vi "RonLinear.vi"(0 "refnum":refnum<file>) -> (4 "refnum out":refnum<file>, 6 "# lines per scan":i32, 8 "sample rate":u16, 10 "# rf points per line":u16, 13 "Scan Settings":T1 {"prf (kHz)" format="%.2f"; "Gain (db)" items=["26.0", "40.0", "54.0"]; "LP Filt (MHz)" items=["20", "50", "100", "200"]; "HP Filt(KHz)" items=["1", "1000", "3000", "10000"]; "Damping (In Ohm)" items=["7", "10", "16", "20", "26", "30", "40", "50"]; "Energy (microJ)" items=["1", "2", "4", "8", "16", "32"]}, 14 "Patient Info":T2={"ID"="", "extended ID"="", "age"=0, "sex"="", "previously\nscanned"="N", "PSA"=0.0, "LOS"=1, "Ethnicty"=3} {"Ethnicty" items=["Am Ind or Alaska", "Asian, Pac Islander", "Black, not Hispanic", "Hispanic", "White, not hispanic", "other, unknown"]; "LOS" items=["1", "2", "3", "4", "5"]; "PSA" format="%.1f"}, 15 "A/D info":T3={"# rf points per line"=0, "# lines per scan"=0, "sample rate MHz"=0, "# A/D bits"=8, "# bytes per A/D"=1, "TGC Flag"=0, "A/D Type"=""})   [LabVIEW 2022 SP3]
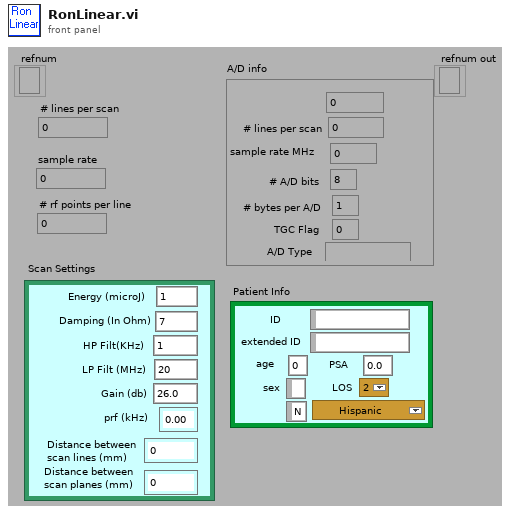
[diagram p1: front panel]
types:
  T1 = cluster{"Energy (microJ)":u8, "Damping (In Ohm)":u8, "HP Filt(KHz) ":u8, "LP Filt (MHz)":u8, "Gain (db)":u8, "prf (kHz)":sgl, "Distance between\nscan lines (mm)":u16, "Distance between\nscan planes (mm)":u16}
  T2 = cluster{"ID":string, "extended ID":string, "age":u16, "sex":string, "previously\nscanned":string, "PSA":sgl, "LOS":u8, "Ethnicty":u8}
  T3 = cluster{"# rf points per line":u16, "# lines per scan":u16, "sample rate MHz":u16, "# A/D bits":i16, "# bytes per A/D":u16, "TGC Flag":u16, "A/D Type":string}
  T4 = cluster{"Energy (microJ)":u8, "Damping (In Ohm)":u8, "HP Filt(KHz)":u8, "LP Filt (MHz)":u8, "Gain (db)":u8, "prf (kHz)":sgl, "Distance between\nscan lines (mm)":u16, "Distance between\nscan planes (mm)":u16}
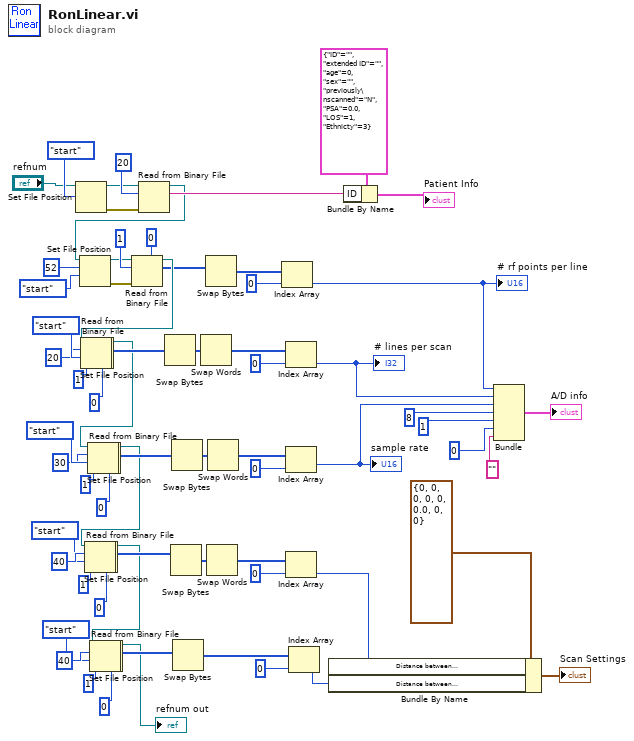
[diagram p0: block diagram]
diagram:
  n1 = Set File Position(refnum="refnum", from (0:start)=enum16{"start", "end", "current"}."start" ("pos mode (0:2)")) -> (refnum out=w7:refnum<file>, error out=w6:errorcluster)  [unwired: 1 in, 1 out]
  n2 = Read from Binary File(8:w6, 10:20, 11:w7) -> (2:w52:string, 3:w44:refnum<file>)  [unwired: 5 out]
  n3 = Set File Position(offset (in bytes) (0)=52 ("pos offset (0)"), refnum=w44, from (0:start)=enum16{"start", "end", "current"}."start" ("pos mode (0:2)")) -> (refnum out=w9:refnum<file>, error out=w8:errorcluster)  [unwired: 1 in]
  n4 = Read from Binary File(5:i16 0, 8:w8, 10:1 ("count"), 11:w9) -> (2:w42:i16[], 3:w43:refnum<file>)  [unwired: 4 out]
  n5 = Set File Position(offset (in bytes) (0)=20 ("pos offset (0)"), refnum=w43, from (0:start)=enum16{"start", "end", "current"}."start" ("pos mode (0:2)")) -> (refnum out=w3:refnum<file>, error out=w2:errorcluster)  [unwired: 1 in]
  n6 = Read from Binary File(5:0, 8:w2, 10:1 ("count"), 11:w3) -> (2:w71:i32[], 3:w58:refnum<file>)  [unwired: 4 out]
  n7 = Set File Position(offset (in bytes) (0)=30 ("pos offset (0)"), refnum=w58, from (0:start)=enum16{"start", "end", "current"}."start" ("pos mode (0:2)")) -> (refnum out=w5:refnum<file>, error out=w4:errorcluster)  [unwired: 1 in]
  n8 = Read from Binary File(5:0, 8:w4, 10:1 ("count"), 11:w5) -> (2:w63:i32[], 3:w33:refnum<file>)  [unwired: 4 out]
  n9 = Set File Position(offset (in bytes) (0)=40 ("pos offset (0)"), refnum=w33, from (0:start)=enum16{"start", "end", "current"}."start" ("pos mode (0:2)")) -> (refnum out=w11:refnum<file>, error out=w10:errorcluster)  [unwired: 1 in]
  n10 = Read from Binary File(5:0, 8:w10, 10:1 ("count"), 11:w11) -> (2:w28:i32[], 3:w19:refnum<file>)  [unwired: 4 out]
  n11 = Set File Position(offset (in bytes) (0)=40 ("pos offset (0)"), refnum=w19, from (0:start)=enum16{"start", "end", "current"}."start" ("pos mode (0:2)")) -> (refnum out=w13:refnum<file>, error out=w12:errorcluster)  [unwired: 1 in]
  n12 = Read from Binary File(5:i16 0, 8:w12, 10:1 ("count"), 11:w13) -> (2:w20:i16[], 3:→"refnum out":refnum<file>)  [unwired: 4 out]
  n13 = Swap Bytes(anything=w71) -> (byte swapped=w68:i32[])
  n14 = Swap Bytes(anything=w28) -> (byte swapped=w30:i32[])
  n15 = Swap Bytes(anything=w63) -> (byte swapped=w60:i32[])
  n16 = Swap Bytes(anything=w20) -> (byte swapped=w18:i16[])
  n17 = Swap Words(1:w68) -> (0:w67:i32[])
  n18 = Swap Bytes(anything=w42) -> (byte swapped=w40:i16[])
  n19 = Swap Words(1:w30) -> (0:w29:i32[])
  n20 = Swap Words(1:w60) -> (0:w59:i32[])
  n21 = Index Array(array=w40, index=0) -> (element=w14:i16)
  "# rf points per line" <- w14
  n22 = Index Array(array=w67, index=0) -> (element=w56:i32)
  "# lines per scan" <- w56
  n23 = Index Array(array=w59, index=0) -> (element=w57:i32)
  "sample rate" <- w57
  n24 = Index Array(array=w29, index=0) -> (element=w16:i32)
  n25 = Index Array(array=w18, index=0) -> (element=w17:i16)
  n26 = Bundle By Name(cluster=T4 {"Energy (microJ)"=0, "Damping (In Ohm)"=0, "HP Filt(KHz)"=0, "LP Filt (MHz)"=0, "Gain (db)"=0, "prf (kHz)"=0.0, "Distance between\nscan lines (mm)"=0, "Distance between\nscan planes (mm)"=0} ("Scan Settings"), "Distance between\nscan planes (mm)"=w16, "Distance between\nscan lines (mm)"=w17) -> (→"Scan Settings":T4)
  n27 = Bundle By Name(cluster=T2 {"ID"="", "extended ID"="", "age"=0, "sex"="", "previously\nscanned"="N", "PSA"=0.0, "LOS"=1, "Ethnicty"=3} ("Patient Info"), "ID"=w52) -> (→"Patient Info":T2)
  n28 = Bundle(w14, w56, w57, 8, 1, 0, "") -> (→"A/D info":cluster{i16, i32, i32, i32, i32, i32, string})  [unwired: 1 out]
